vi "Helper - UTM To Image.vi"(3 "error in":errorcluster, 4 "Image Descriptor":T2={"Upper-Left Corner Coordinates"={"UTM Zone"=0.0, "Hemisphere"=enum."North", "East"=0.0, "North"=0.0}, "Meters/Pixel"=42.294203} {"Upper-Left Corner Coordinates"."North" format="%#_10f"; "Upper-Left Corner Coordinates"."East" format="%#_8f"}, 5 "UTM Location":T1 {"North" format="%#_10f"; "East" format="%#_8f"}) -> (0 "error out":errorcluster, 1 "Coordinate Outside Image":bool, 2 "Pixel Coordinates":cluster{"X":i32, "Y":i32})   [LabVIEW 2011]
uses:
  0-OCU/0 Code/mission input/0-Image Descriptor.ctl
  2 Typedefs/UTM Location.ctl
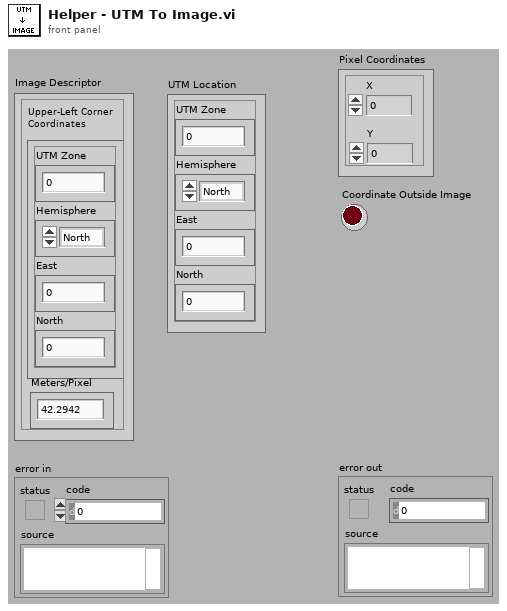
[diagram p1: front panel]
types:
  T1 = typedef "UTM Location.ctl" = cluster{"UTM Zone":dbl, "Hemisphere":enum16{"North", "South"}, "East":dbl, "North":dbl}
  T2 = typedef "0-Image Descriptor.ctl" = cluster{"Upper-Left Corner Coordinates":T1, "Meters/Pixel":dbl}
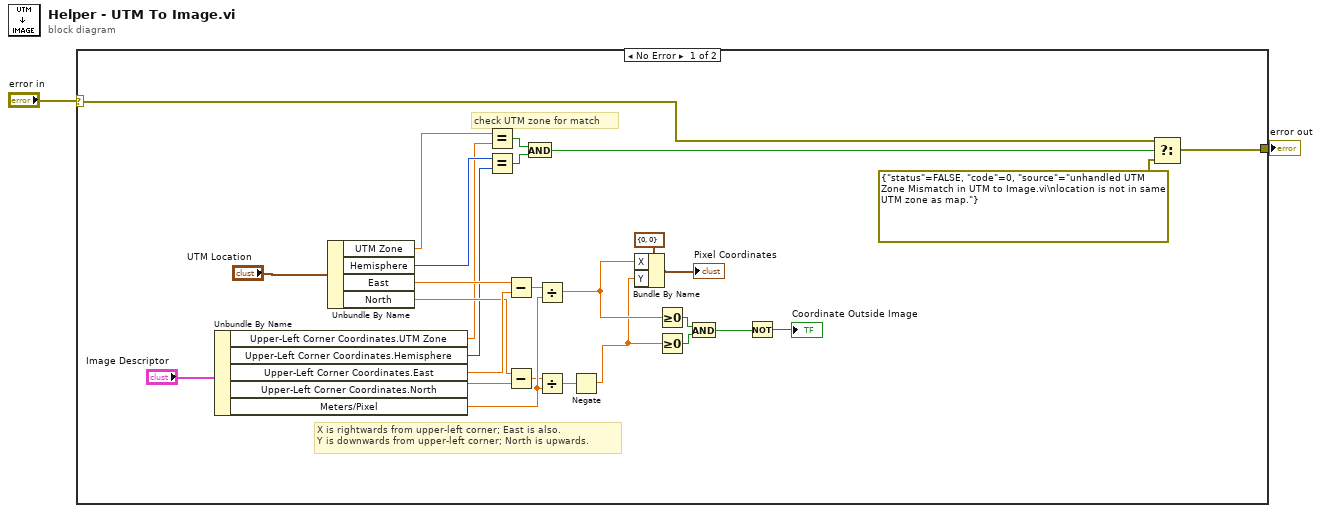
[diagram p0: block diagram]
diagram:
  n1 = case shown="No Error" "error in" {
    selector: "error in" -> [w8 w31]
    tunnel: [w12 w31] -> w1
    frame No Error {
      # "check UTM zone for match"
      # "X is rightwards from upper-left corner; East is also.\nY is downwards from upper-left corner; North is upwards."
      n2 = Unbundle By Name("Image Descriptor") -> ("Upper-Left Corner Coordinates.UTM Zone"=w18:dbl, "Upper-Left Corner Coordinates.Hemisphere"=w19:enum16{"North", "South"}, "Upper-Left Corner Coordinates.East"=w28:dbl, "Upper-Left Corner Coordinates.North"=w27:dbl, "Meters/Pixel"=w26:dbl)
      n3 = Unbundle By Name("UTM Location") -> ("UTM Zone"=w17:dbl, "Hemisphere"=w20:enum16{"North", "South"}, "East"=w23:dbl, "North"=w22:dbl)
      n4 = Equal?(x=w17, y=w18) -> (x = y?=w16:bool)
      n5 = Equal?(x=w20, y=w19) -> (x = y?=w15:bool)
      n6 = Subtract(x=w23, y=w28) -> (x-y=w21:dbl)
      n7 = Subtract(x=w22, y=w27) -> (x-y=w25:dbl)
      n8 = And(x=w16, y=w15) -> (x .and. y?=w14:bool)
      n9 = Divide(x=w21, y=w26) -> (x/y=w5:dbl)
      n10 = Divide(x=w25, y=w26) -> (x/y=w30:dbl)
      n11 = Negate(x=w30) -> (-x=w4:dbl)
      n12 = Bundle By Name(cluster=cluster{"X":i32, "Y":i32} {"X"=0, "Y"=0} ("Pixel Coordinates 2"), "X"=w5, "Y"=w4) -> (→"Pixel Coordinates":cluster{"X":i32, "Y":i32})
      n13 = Greater Or Equal To 0?(x=w5) -> (x >= 0?=w10:bool)
      n14 = Greater Or Equal To 0?(x=w4) -> (x >= 0?=w11:bool)
      n15 = And(x=w10, y=w11) -> (x .and. y?=w9:bool)
      n16 = Not(x=w9) -> (.not. x?=→"Coordinate Outside Image":bool)
      n17 = Select(t=w8, s=w14, f=errorcluster {"status"=FALSE, "code"=0, "source"="unhandled UTM Zone Mismatch in UTM to Image.vi\nlocation is not in same UTM zone as map."} ("error IO")) -> (s? t:f=w12:errorcluster)
    }
    frame Error {
    }
  }
  "error out" <- w1
